vi "get_coordinates.vi"(8 "error in (no error)":errorcluster, 11 "GenericTrajectory in":refnum<class "TrajectoryDL091126GenericVoxel.lvclass">) -> (0 "error out":errorcluster, 2 "coordinates":dbl[unit][][](array[numeric]), 3 "GenericTrajectory out":refnum<class "TrajectoryDL091126GenericVoxel.lvclass">)   [LabVIEW 2010, in "TrajectoryDL091126GenericVoxel.lvclass"]
uses:
  TrajectoryDL091126GenericVoxel.lvclass
  common/enumerations/x_y_z_enumeration.ctl
  common/enumerations/functional_global_action_enum.ctl
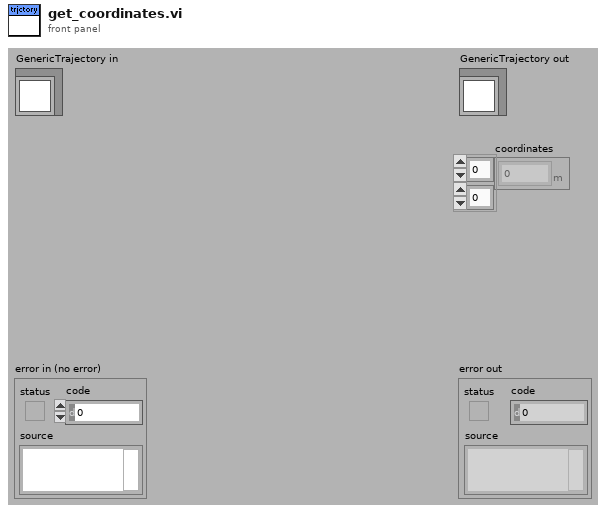
[diagram p1: front panel]
types:
  T1 = typedef "x_y_z_enumeration.ctl" = enum16{"x", "y", "z"}
  T2 = typedef "functional_global_action_enum.ctl" = enum16{"get", "set", "reset"}
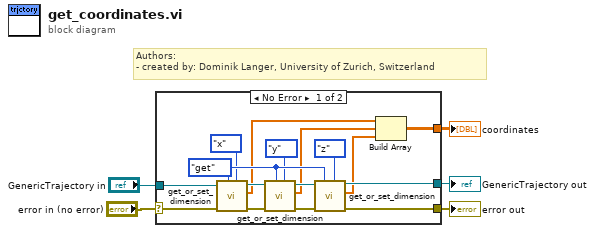
[diagram p0: block diagram]
diagram:
  # "Authors: \n- created by: Dominik Langer, University of Zurich, Switzerland"
  n1 = case shown="No Error" "error in (no error)" {
    selector: "error in (no error)" -> [w15 w23]
    tunnel: [w14 w23] -> w4
    tunnel: [w12 w22] -> w2
    tunnel: "GenericTrajectory in" -> [w13 w22]
    tunnel: [w21 _] -> w1
    frame No Error {
      w20 = functional_global_action_enum."get" ("action")
      n2 = call-dynamic "get_or_set_dimension.vi"("dimension"=x_y_z_enumeration."x", "action"=w20, "error in (no error)"=w15, "GenericTrajectory in"=w13) -> ("error out"=w17:errorcluster, "pixel values out (single dimension)"=w11:dbl[unit][], "GenericTrajectory out"=w18:refnum<class "TrajectoryDL091126GenericVoxel.lvclass">)  [unwired: 2 in, 3 out]
      n3 = call-dynamic "get_or_set_dimension.vi"("dimension"=x_y_z_enumeration."y", "action"=w20, "error in (no error)"=w17, "GenericTrajectory in"=w18) -> ("error out"=w16:errorcluster, "pixel values out (single dimension)"=w10:dbl[unit][], "GenericTrajectory out"=w19:refnum<class "TrajectoryDL091126GenericVoxel.lvclass">)  [unwired: 2 in, 3 out]
      n4 = call-dynamic "get_or_set_dimension.vi"("dimension"=x_y_z_enumeration."z", "action"=w20, "error in (no error)"=w16, "GenericTrajectory in"=w19) -> ("error out"=w14:errorcluster, "pixel values out (single dimension)"=w9:dbl[unit][], "GenericTrajectory out"=w12:refnum<class "TrajectoryDL091126GenericVoxel.lvclass">)  [unwired: 2 in, 3 out]
      n5 = Build Array(w11, w10, w9) -> (w21:dbl[unit][][])
    }
    frame Error {
    }
  }
  "error out" <- w4
  "GenericTrajectory out" <- w2
  "coordinates" <- w1
